vi "Handle Last Ack Core.vi"(4 "error in (no error)":errorcluster, 6 "Last Ack":refnum<class "Last Ack.lvclass">, 7 "Actor Example in":refnum<class "Actor Example.lvclass">) -> (0 "error out":errorcluster, 3 "Actor Example out":refnum<class "Actor Example.lvclass">)   [LabVIEW 2017, in "Actor Example.lvlib" / "Actor Example.lvclass"]
doc: "(<B>Filename</B>: Actor Framework.lvlib:Actor.lvclass:Handle Last Ack Core.vi)\n\nDefines how the caller actor responds to the Last Ack message from a nested actor. The Last Ack message is the final message a nested actor sends to its caller before it shuts down. The message contains information about the final state of the nested actor.\n\nBy default, this method does nothing except return any error the nested actor sent. A descendant class may override this method to define behavior."
uses:
  Actor Example.lvclass
  <vilib>/ActorFramework/LastAck/Last Ack.lvclass
  C:/Program Files (x86)/National Instruments/LabVIEW 2017/vi.lib/ActorFramework/Actor/Actor.lvclass
  Long Running Process/Long Running Process.lvclass
  Promise Future/Promise/Promise.lvclass
  E:/Promise/Promise Future/Future/Future.lvclass
  <vilib>/ActorFramework/LastAck/Last Ack.lvclass/Last Ack.ctl
  Long Running Process/Long Running Process.lvclass/Long Running Process.ctl
  <vilib>/ActorFramework/Actor/Actor.lvclass/Actor.ctl
  <vilib>/ActorFramework/Message Enqueuer/Message Enqueuer.lvclass/Message Enqueuer.ctl
  Actor Example.lvclass/Actor Example.ctl
  Actor Example Messages/Start Long Running Process Msg/Start Long Running Process Msg.lvclass/Start Long Running Process Msg.ctl
  6fa8b397-9bbc-4ad2-8fcf-cf3c44e803f2.vi
  8f9d7b8a-72c1-4d90-96cd-587bc6981dfa.vi
  Long Running Process/Read Result.vi
  <vilib>/ActorFramework/Message Enqueuer/Init from Existing Queue.vi
  <vilib>/ActorFramework/Message Enqueuer/Enqueue.vi
  Actor Example Messages/Start Long Running Process Msg/Start Long Running Process Msg.lvclass
  C:/Program Files (x86)/National Instruments/LabVIEW 2017/vi.lib/ActorFramework/Message/Message.lvclass
  <vilib>/Utility/error.llb/Error Cluster From Error Code.vi
  Promise Future/Promise/Obtain Promise.vi
  Promise Future/Promise/Read Future.vi
  <vilib>/ActorFramework/Message Priority Queue/Priority Enqueue.vi
  Promise Future/Future/Write Future.vi
  <vilib>/MGI/Monitored Actor/Monitored Actor/Monitored Actor/Monitored Actor.lvclass
  <vilib>/ActorFramework/Message Enqueuer/Message Enqueuer.lvclass
  <vilib>/ErrorRing/Error Ring.xnode
  <vilib>/ActorFramework/Actor/Actor.lvclass
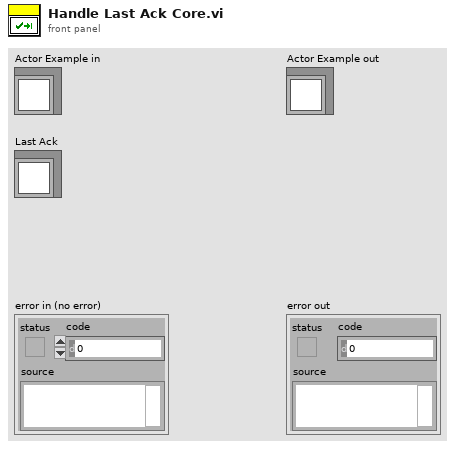
[diagram p1: front panel]
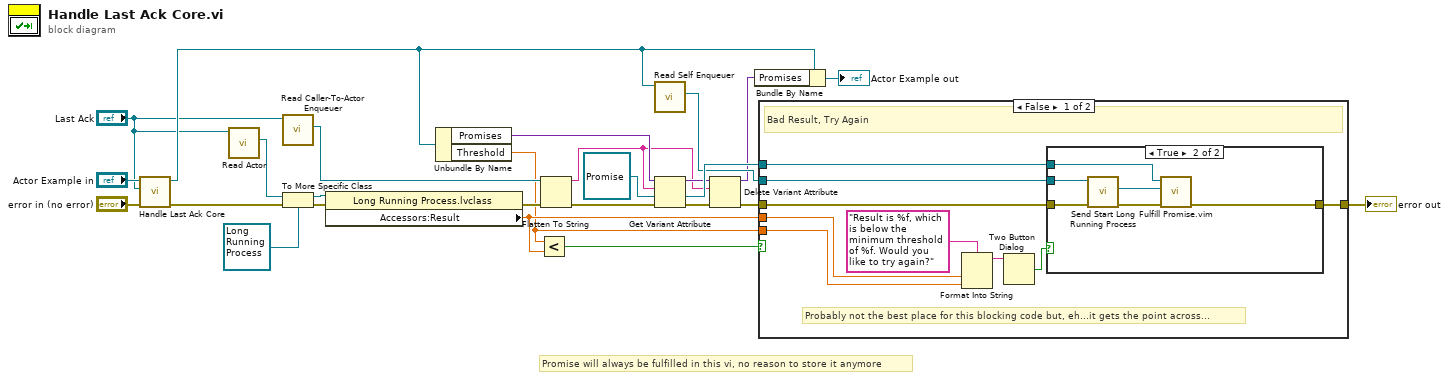
[diagram p0: block diagram]
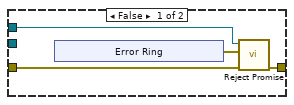
[diagram p2: hidden frame]
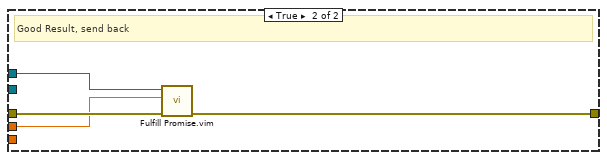
[diagram p3: hidden frame]
diagram:
  # "Promise will always be fulfilled in this vi, no reason to store it anymore"
  n1 = call-parent "Handle Last Ack Core.vi"("error in (no error)"="error in (no error)", "Last Ack"="Last Ack", "Actor in"="Actor Example in") -> ("error out"=w3:errorcluster, "Actor out"=w5:refnum<class "Actor Example.lvclass">)  [unwired: 3 in]
  n2 = call <vilib>:"Read Actor.vi"("Last Ack"="Last Ack") -> ("Actor"=w26:refnum<class "Actor.lvclass">)  [unwired: 10 in]
  n3 = call <vilib>:"Read Caller-To-Actor Enqueuer.vi"("Last Ack"="Last Ack") -> ("Caller-to-Actor Enqueuer"=w22:refnum<class "Message Enqueuer.lvclass">)  [unwired: 10 in]
  n4 = To More Specific Class(target class=refnum<class "Long Running Process.lvclass"> refnum ("Actor Example.lvlib:Long Running Process.lvclass"), reference=w26, error in=w3) -> (specific class reference=w25:refnum<class "Long Running Process.lvclass">, error out=w15:errorcluster)
  n5 = property class="Long Running Process.lvclass"(reference=w25, error in=w15) -> (error out=w14:errorcluster, "Accessors:Result"=w19:dbl)  [unwired: 1 out]
  n6 = Unbundle By Name(w5) -> ("Promises"=w23:variant, "Threshold"=w9:dbl)
  n7 = Less?(x=w9, y=w19) -> (x < y?=w20:bool)
  n8 = Flatten To String(anything=w22, error in (no error)=w14) -> (data string=w16:string, error out=w13:errorcluster)  [unwired: 2 in, 1 out]
  n9 = call <vilib>:"Read Self Enqueuer.vi"("Actor"=w5) -> ("Self Enqueuer"=w18:refnum<class "Message Enqueuer.lvclass">)  [unwired: 10 in]
  n10 = Get Variant Attribute(Variant=w23, name=w16, default value (empty Variant)=refnum<class "Promise.lvclass"> refnum ("Promise Future.lvlib:Promise.lvclass"), error in=w13) -> (duplicate Variant=w17:variant, value=w21:refnum<class "Promise.lvclass">, error out=w12:errorcluster)  [unwired: 1 out]
  n11 = Delete Variant Attribute(4:w12, 6:w16, 7:w17) -> (0:w11:errorcluster, 3:w10:variant)  [unwired: 1 out]
  n12 = Bundle By Name(cluster=w5, "Promises"=w10) -> (→"Actor Example out":refnum<class "Actor Example.lvclass">)
  n13 = case shown="False" w20 {
    tunnel: w21 -> [w35 w51]
    tunnel: w19 -> [w29 w52]
    tunnel: w18 -> [w34 _]
    tunnel: w11 -> [w33 w53]
    tunnel: [w32 w54] -> w7
    tunnel: w9 -> [w28 _]
    frame False {
      # "Probably not the best place for this blocking code but, eh...it gets the point across..."
      # "Bad Result, Try Again"
      n14 = Format Into String(format string="Result is %f, which is below the minimum threshold of %f. Would you like to try again?", w29, w28) -> (resulting string=w30:string)  [unwired: 2 in, 1 out]
      n15 = Two Button Dialog(message=w30) -> (T button?=w31:bool)  [unwired: 2 in]
      n16 = case shown="True" w31 {
        tunnel: w35 -> [w38 w45]
        tunnel: w34 -> [_ w50]
        tunnel: w33 -> [w39 w49]
        tunnel: [w36 w47] -> w32
        frame False {
          n17 = xnode "Error Ring"() -> ("error out"=w37:errorcluster)
          n18 = call "Reject Promise.vi"("error in (no error)"=w39, "Reason"=w37, "Promise in"=w38) -> ("error out"=w36:errorcluster)  [unwired: 7 in, 1 out]
        }
        frame True {
          n19 = call "Send Start Long Running Process.vi"("error in (no error)"=w49, "Message Enqueuer"=w50) -> ("error out"=w48:errorcluster, "Future"=w46:refnum<class "Future.lvclass">)  [unwired: 7 in, 1 out]
          n20 = call "Fulfill Promise.vim"("error in (no error)"=w48, "Value"=w46, "Promise in"=w45) -> ("error out"=w47:errorcluster)  [unwired: 7 in, 1 out]
        }
      }
    }
    frame True {
      # "Good Result, send back"
      n21 = call "Fulfill Promise.vim"("error in (no error)"=w53, "Value"=w52, "Promise in"=w51) -> ("error out"=w54:errorcluster)  [unwired: 7 in, 1 out]
    }
  }
  "error out" <- w7
